vi "Attached Camera AE.vi"(7 "Update":bool, 11 "Camera List in":string[](array[string])=["cam0"]) -> (3 "Camera List out":string[](array[string])=["cam0"])   [LabVIEW 2023]
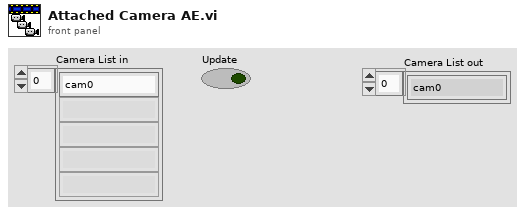
[diagram p1: front panel]
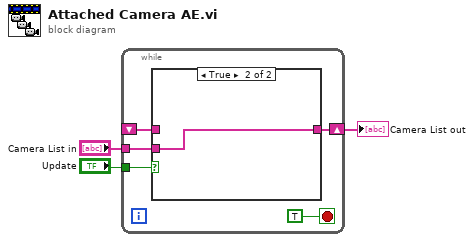
[diagram p0: block diagram]
diagram:
  n1 = while {
    tunnel: "Update" -> [w7]
    shift-right: [w5] -> w2
    shift-left: _ -> [w6]
    tunnel: "Camera List in" -> [w4]
    stop <- TRUE stop-if-true
    n2 = case shown="True" w7 {
      tunnel: w6 -> [w9 _]
      tunnel: [w9 w10] -> w5
      tunnel: w4 -> [_ w10]
      frame False {
      }
      frame True {
      }
    }
  }
  "Camera List out" <- w2
